vi "CP Removal.vi"(0 "Input":cdb[](array[numeric]), 7 "Indicies":i32, 11 "i":i32, 12 "Frame Size":i32, 13 "CP Size":i32, 14 "N-Point FFT Size":i32) -> (4 "Output Without CP":cdb[](array[numeric]))   [LabVIEW 2022 SP3]
doc: "Removes cyclix prefix (CP) from a frame and extracts N-point data symbols\nFrame=CP+DATA"
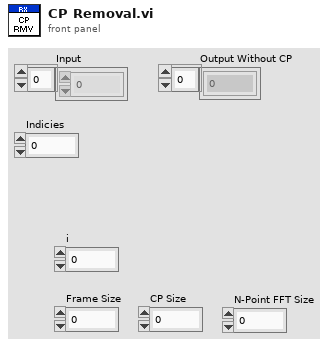
[diagram p1: front panel]
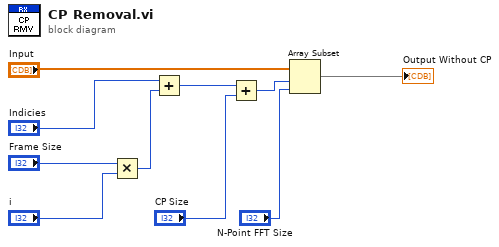
[diagram p0: block diagram]
diagram:
  n1 = Multiply(x="Frame Size", y="i") -> (x*y=w5:i32)
  n2 = Add(x="Indicies", y=w5) -> (x+y=w4:i32)
  n3 = Add(x=w4, y="CP Size") -> (x+y=w3:i32)
  n4 = Array Subset(array="Input", index=w3, length="N-Point FFT Size") -> (→"Output Without CP":cdb[])
